vi "ConfigClkRef.vi"(8 "error in (no error)":errorcluster, 11 "PXI_MultiTrig in":refnum<class "PXI_MultiTrig.lvclass">) -> (0 "error out":errorcluster, 3 "PXI_MultiTrig out":refnum<class "PXI_MultiTrig.lvclass">)   [LabVIEW 2014, in "SyncPlugins.lvlib" / "PXI_MultiTrig.lvclass"]
uses:
  PXI_MultiTrig.lvclass
  PXI_MultiTrig.lvclass/PXI_MultiTrig.ctl
  Accessors/Read TimeRefType.vi
  Accessors/Read RefClkHandle.vi
  Accessors/Write RefClkSession.vi
  <instrlib>/niSync/niSync.llb/niSync Initialize (IVI).vi
  <instrlib>/niSync/niSync.llb/niSync Set Time Reference (1588 Ordinary Clock).vi
  <instrlib>/niSync/niSync.llb/niSync Set Time Reference (Free Running).vi
  <instrlib>/niSync/niSync.llb/niSync Set Time Reference (GPS).vi
  <instrlib>/niSync/niSync.llb/niSync Set Time Reference (IRIG).vi
  <instrlib>/niSync/niSync.llb/niSync Set Time Reference (PPS).vi
panel:
  out "Timing:GPS:Status":i32(ring) items=["Uninitialized", "Antenna Error", "No Useable Satellites", "One Useable Satellite", "Two Useable Satellites", "Three Useable Satellites", "No GPS Time", "PDOP Too High", "Unusable Satellite", "Fix Rejected", "Self Survey Complete", "Self Survey Not Complete"]
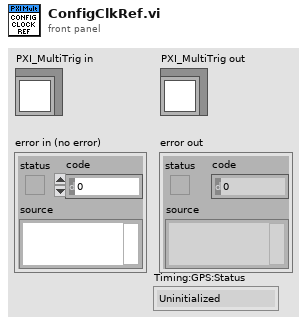
[diagram p1: front panel]
types:
  T1 = typedef "SyncPlugins.lvlib/PXI_MultiTrig.lvclass/TimeRefType.ctl" = enum16{"1588", "Free Running", "GPS", "IRIG", "PPS"}
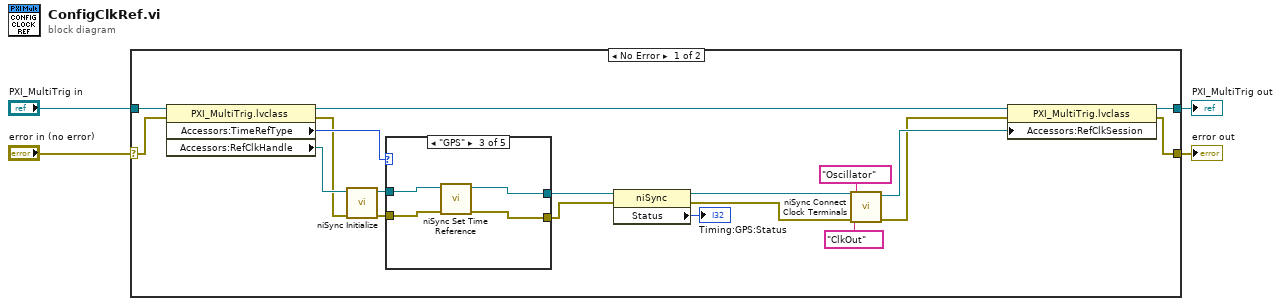
[diagram p0: block diagram]
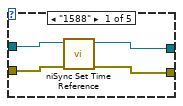
[diagram p2: hidden frame]
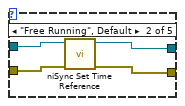
[diagram p3: hidden frame]
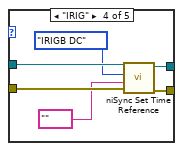
[diagram p4: hidden frame]
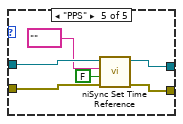
[diagram p5: hidden frame]
diagram:
  n1 = case shown="No Error" "error in (no error)" {
    selector: "error in (no error)" -> [w21 w49]
    tunnel: [w20 w49] -> w3
    tunnel: [w22 w48] -> w1
    tunnel: "PXI_MultiTrig in" -> [w23 w48]
    frame No Error {
      n2 = property class="PXI_MultiTrig.lvclass"(reference=w23, error in=w21) -> (reference out=w10:refnum<class "PXI_MultiTrig.lvclass">, error out=w8:errorcluster, "Accessors:TimeRefType"=w17:T1, "Accessors:RefClkHandle"=w18:refnum<k15>)
      n3 = call-poly <instrlib>:"niSync Initialize.vi"("error in (no error)"=w8, "resource name"=w18) -> ("error out"=w13:errorcluster, "instrument handle out"=w16:refnum<k15>)  [unwired: 8 in]
      n4 = case shown="\"GPS\"" w17 {
        tunnel: w16 -> [w27 w31 w35 w41 w47]
        tunnel: w13 -> [w26 w30 w34 w40 w46]
        tunnel: [w25 w29 w33 w39 w45] -> w15
        tunnel: [w24 w28 w32 w38 w44] -> w7
        frame "1588" {
          n5 = call-poly <instrlib>:"niSync Set Time Reference.vi"("error in (no error)"=w26, "instrument handle"=w27) -> ("error out"=w24:errorcluster, "instrument handle out"=w25:refnum<k15>)  [unwired: 8 in]
        }
        frame "Free Running", Default {
          n6 = call-poly <instrlib>:"niSync Set Time Reference.vi"("error in (no error)"=w30, "instrument handle"=w31) -> ("error out"=w28:errorcluster, "instrument handle out"=w29:refnum<k15>)  [unwired: 8 in]
        }
        frame "GPS" {
          n7 = call-poly <instrlib>:"niSync Set Time Reference.vi"("error in (no error)"=w34, "instrument handle"=w35) -> ("error out"=w32:errorcluster, "instrument handle out"=w33:refnum<k15>)  [unwired: 8 in]
        }
        frame "IRIG" {
          n8 = call-poly <instrlib>:"niSync Set Time Reference.vi"("error in (no error)"=w40, "terminal"=tag "", "IRIG type"=enum16{"IRIGB DC", "IRIGB AM"}."IRIGB DC", "instrument handle"=w41) -> ("error out"=w38:errorcluster, "instrument handle out"=w39:refnum<k15>)  [unwired: 6 in]
        }
        frame "PPS" {
          n9 = call-poly <instrlib>:"niSync Set Time Reference.vi"("error in (no error)"=w46, "use manual time"=FALSE, "terminal"=tag "", "instrument handle"=w47) -> ("error out"=w44:errorcluster, "instrument handle out"=w45:refnum<k15>)  [unwired: 6 in]
        }
      }
      n10 = property class="niSync"(reference=w15, error in=w7) -> (reference out=w9:refnum<k15>, error out=w6:errorcluster, "Status"=→"Timing:GPS:Status":i32)
      n11 = call <instrlib>:"niSync Connect Clock Terminals.vi"("error in (no error)"=w6, "destination terminal"="ClkOut", "source terminal"="Oscillator", "instrument handle"=w9) -> ("error out"=w11:errorcluster, "instrument handle out"=w12:refnum<k15>)  [unwired: 6 in]
      n12 = property class="PXI_MultiTrig.lvclass"(reference=w10, error in=w11, "Accessors:RefClkSession"=w12) -> (reference out=w22:refnum<class "PXI_MultiTrig.lvclass">, error out=w20:errorcluster)
    }
    frame Error {
    }
  }
  "error out" <- w3
  "PXI_MultiTrig out" <- w1
